vi "flow meter test.vi"() -> ()   [LabVIEW 2019]
uses:
  <vilib>/FPGAPlugInAG/sbRIO-9626/niLvFpga_Open_sbRIO-9626.vi
  <vilib>/rvi/interface/common/dynamic/niFpgaDynamicAddResources.vi
  <vilib>/Utility/error.llb/Error Cluster From Error Code.vi
  <vilib>/rvi/errors/niLvFpgaAdjustHostInterfaceError.vi
  <vilib>/rvi/interface/nirviOpenFPGA/nirviOpenFPGA.xnode
  FPGA/bitfiles/Flow Meter Test.lvbitx
  <vilib>/rvi/interface/nirviReadWriteControl/nirviReadWriteControl.xnode
  NiFpgaLv.dll
  <vilib>/rvi/interface/Simulation/niFpgaSimulationCallBeginRW.vi
panel:
  out "Frequency":dbl[](array[numeric])
  out "Period":u32[](array[numeric])
  out "Waveform Chart":T1(graph)
  in  "stop":bool
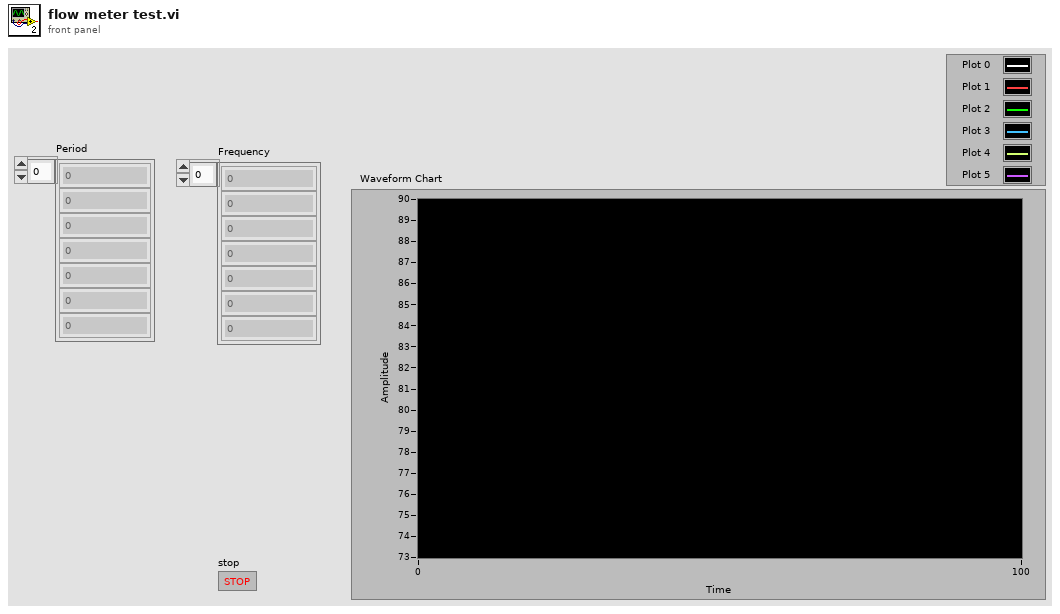
[diagram p1: front panel]
types:
  T1 = cluster{"[0]":dbl, "[1]":dbl, "[2]":dbl, "[3]":dbl, "[4]":dbl, "[5]":dbl, "[6]":dbl, "[7]":dbl, "[8]":dbl}
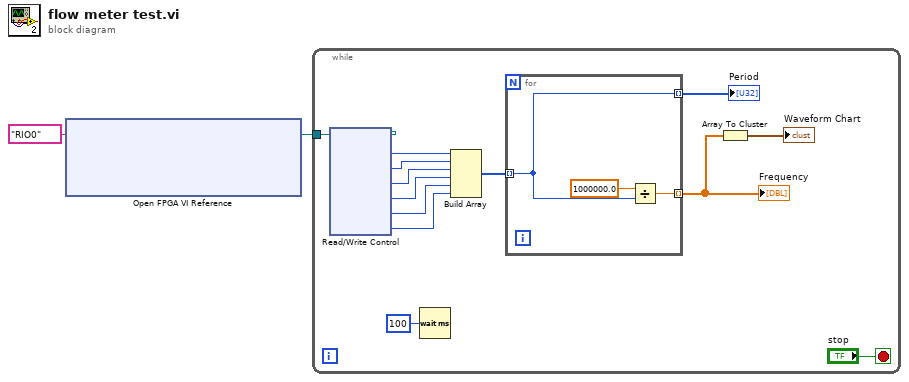
[diagram p0: block diagram]
diagram:
  n1 = xnode "Open FPGA VI Reference"("resource name"=tag "RIO0") -> ("FPGA VI Reference Out"=w2:refnum<k20>)  [unwired: 1 in, 1 out]
  n2 = while {
    tunnel: w2 -> [w14]
    stop <- "stop" stop-if-true
    n3 = xnode "Read/Write Control"("FPGA VI Reference In"=w14) -> ("Period 1"=w12:u32, "Period 2"=w11:u32, "Period 3"=w10:u32, "Period 4"=w9:u32, "Period 5"=w8:u32, "Period 6"=w7:u32)  [unwired: 1 in, 2 out]
    n4 = Wait (ms)(milliseconds to wait=u32 100) -> ()  [unwired: 1 out]
    n5 = Build Array(w12, w11, w10, w9, w8, w7) -> (w6:u32[])
    n6 = for {
      tunnel: [w16] -> w4 mode=indexing
      tunnel: [w17] -> w5 mode=indexing
      tunnel: w6 -> [w16] mode=indexing
      n7 = Divide(x=1000000.0, y=w16) -> (x/y=w17:dbl)
    }
    "Frequency" <- w5
    "Period" <- w4
    n8 = Array To Cluster(array=w5) -> (cluster=→"Waveform Chart":T1)
  }
